vi "Find Length.vi"(8 "error in (no error)":errorcluster, 10 "IK Parameters":T2, 11 "Data in":T1={"link 1 angle"=0.0, "link 2 angle"=0.0, "link 1 length"=0.0, "link 2 length"=0.0, "Current arm location"=[{"X"=0.0, "Y"=0.0}, {"X"=-37.249783598972314, "Y"=33.353464914904016}, {"X"=-74.49956719794463, "Y"=66.70692982980803}], "Link Picture"=bytes[1162], "Desired Location"={"Desired X"=0.0, "Desired Y"=0.0}, "Next Location"={"Next X"=0.0, "Next Y"=0.0}, "Error"={"Joint1 error"=0.0, "Joint2 error"=0.0}, "tdms data"=refnum, "de/dt"={"joint1 de/dt"=0.0, "joint2 de/dt"=0.0}, "Voltages"={"Joint1 voltage"=0.0, "Joint2 voltage"=0.0}, "Time"=0.0, "dt"=0.0, "counts/rev"=0.0, "kp"=0.0, "kd"=0.0, "ki"=0.0, "Int(error)"={"joint1 int(e)"=0.0, "joint2 int(e)"=0.0}, "Desired angles"={"theta 1"=0.0, "theta 2"=0.0}, "Current counts"={"theta 1"=0.0, "theta 2"=0.0}, "Desired Counts"={"theta 1"=0.0, "theta 2"=0.0}, "Preivous Error"={"Joint1 Previous error"=0.0, "Joint2 Previous error"=0.0}, "Counts/s"=0.0, "Correct counter"=0}) -> (0 "error out":errorcluster, 2 "IK Parameters Out":T2, 3 "Data Out":T1={"link 1 angle"=0.0, "link 2 angle"=0.0, "link 1 length"=0.0, "link 2 length"=0.0, "Current arm location"=[{"X"=0.0, "Y"=0.0}, {"X"=-37.249783598972314, "Y"=33.353464914904016}, {"X"=-74.49956719794463, "Y"=66.70692982980803}], "Link Picture"=bytes[1162], "Desired Location"={"Desired X"=0.0, "Desired Y"=0.0}, "Next Location"={"Next X"=0.0, "Next Y"=0.0}, "Error"={"Joint1 error"=0.0, "Joint2 error"=0.0}, "tdms data"=refnum, "de/dt"={"joint1 de/dt"=0.0, "joint2 de/dt"=0.0}, "Voltages"={"Joint1 voltage"=0.0, "Joint2 voltage"=0.0}, "Time"=0.0, "dt"=0.0, "counts/rev"=0.0, "kp"=0.0, "kd"=0.0, "ki"=0.0, "Int(error)"={"joint1 int(e)"=0.0, "joint2 int(e)"=0.0}, "Desired angles"={"theta 1"=0.0, "theta 2"=0.0}, "Current counts"={"theta 1"=0.0, "theta 2"=0.0}, "Desired Counts"={"theta 1"=0.0, "theta 2"=0.0}, "Preivous Error"={"Joint1 Previous error"=0.0, "Joint2 Previous error"=0.0}, "Counts/s"=0.0, "Correct counter"=0})   [LabVIEW 2016]
uses:
  Type Defs/IK parameters.ctl
  Type Defs/Host Data.ctl
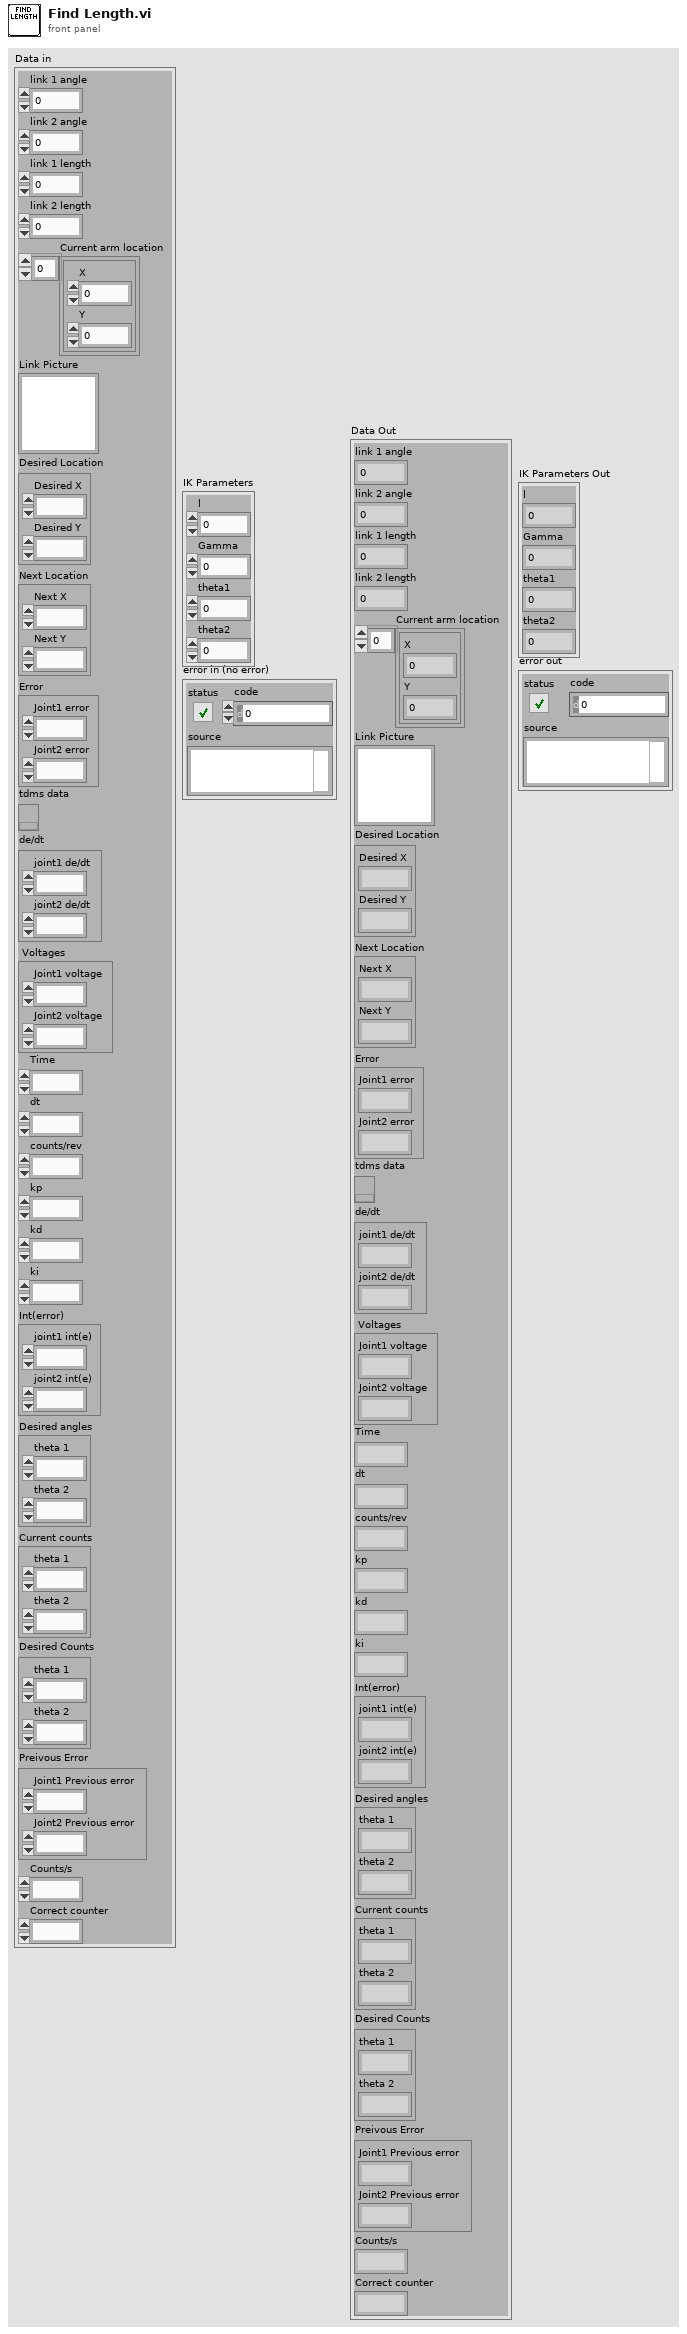
[diagram p1: front panel]
types:
  T1 = typedef "Host Data.ctl" = cluster{"link 1 angle":dbl, "link 2 angle":dbl, "link 1 length":dbl, "link 2 length":dbl, "Current arm location":cluster{"X":dbl, "Y":dbl}[], "Link Picture":picture, "Desired Location":cluster{"Desired X":dbl, "Desired Y":dbl}, "Next Location":cluster{"Next X":dbl, "Next Y":dbl}, "Error":cluster{"Joint1 error":dbl, "Joint2 error":dbl}, "tdms data":refnum<k34>, "de/dt":cluster{"joint1 de/dt":dbl, "joint2 de/dt":dbl}, "Voltages":cluster{"Joint1 voltage":dbl, "Joint2 voltage":dbl}, "Time":dbl, "dt":dbl, "counts/rev":dbl, "kp":dbl, "kd":dbl, "ki":dbl, "Int(error)":cluster{"joint1 int(e)":dbl, "joint2 int(e)":dbl}, "Desired angles":cluster{"theta 1":dbl, "theta 2":dbl}, "Current counts":cluster{"theta 1":dbl, "theta 2":dbl}, "Desired Counts":cluster{"theta 1":dbl, "theta 2":dbl}, "Preivous Error":cluster{"Joint1 Previous error":dbl, "Joint2 Previous error":dbl}, "Counts/s":dbl, "Correct counter":i32}
  T2 = typedef "IK parameters.ctl" = cluster{"l":dbl, "Gamma":dbl, "theta1":dbl, "theta2":dbl}
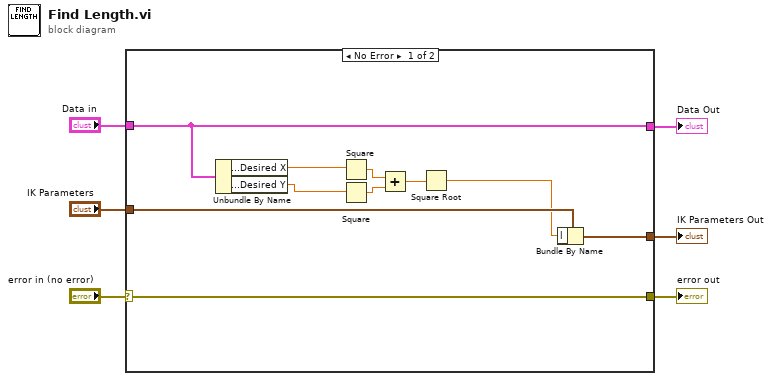
[diagram p0: block diagram]
diagram:
  n1 = case shown="No Error" "error in (no error)" {
    selector: "error in (no error)" -> [w7 w19]
    tunnel: [w7 w19] -> w5
    tunnel: "Data in" -> [w11 w18]
    tunnel: "IK Parameters" -> [w10 w17]
    tunnel: [w11 w18] -> w2
    tunnel: [w8 w17] -> w1
    frame No Error {
      n2 = Unbundle By Name(w11) -> ("Desired Location.Desired X"=w16:dbl, "Desired Location.Desired Y"=w15:dbl)
      n3 = Square(x=w16) -> (x^2=w14:dbl)
      n4 = Square(x=w15) -> (x^2=w13:dbl)
      n5 = Add(x=w14, y=w13) -> (x+y=w12:dbl)
      n6 = Square Root(x=w12) -> (sqrt(x)=w9:dbl)
      n7 = Bundle By Name(cluster=w10, "l"=w9) -> (w8:T2)
    }
    frame Error {
    }
  }
  "error out" <- w5
  "IK Parameters Out" <- w1
  "Data Out" <- w2
